vi "Set_and_Wait.vi"() -> ()   [LabVIEW 2010]
panel:
  in  "Adress":string
  in  "Voltage":dbl
  in  "error in":errorcluster
  out "error out":errorcluster
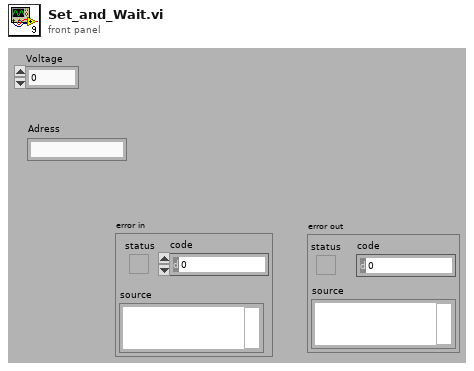
[diagram p1: front panel]
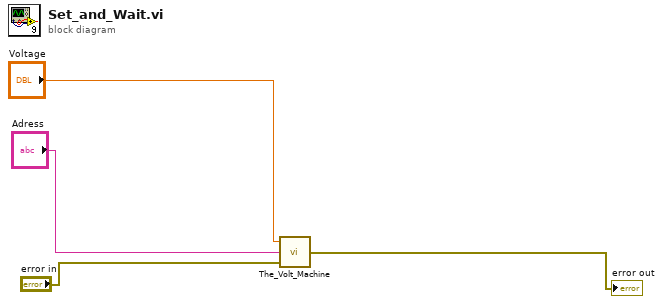
[diagram p0: block diagram]
diagram:
  n1 = call "The_Volt_Machine.vi"("error in"="error in", "Adress"="Adress", "Voltage"="Voltage") -> ("error out"=→"error out":errorcluster)
